vi "test全局.vi"() -> ()   [LabVIEW 2022 SP3]
panel:
  out "quit":bool
  out "st":dbl
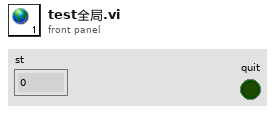
[diagram p1: front panel]
diagram:
